vi "XML Script - GenericSubVI.vi"   [LabVIEW 2020]
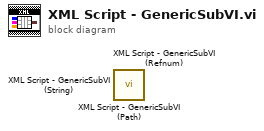
[diagram p0: block diagram]
diagram:
  n1 = call <vilib>:"XML Script - GenericSubVI (Path).vi"() -> ()  [unwired: 8 in, 2 out]
  n2 = call <vilib>:"XML Script - GenericSubVI (Refnum).vi"() -> ()  [unwired: 8 in, 2 out]
  n3 = call <vilib>:"XML Script - GenericSubVI (String).vi"() -> ()  [unwired: 8 in, 2 out]
